vi "Update State Connections.vi"(8 "error in (no error)":errorcluster, 9 "connection list":T1[](array[typedef]), 10 "State":string, 11 "Channel Ref in":T2 format="%.0x") -> (0 "error out":errorcluster, 3 "Channel Ref out":T2=18446744073709551615 format="%.0x")   [LabVIEW 2017, in "Switch Scripting.lvlib"]
uses:
  Switch Scripting.lvlib
  <vilib>/NI Veristand/Custom Device API/Custom Device Item Ref.ctl
  Connection.ctl
  <vilib>/NI VeriStand/Custom Device API/Custom Device API.lvlib
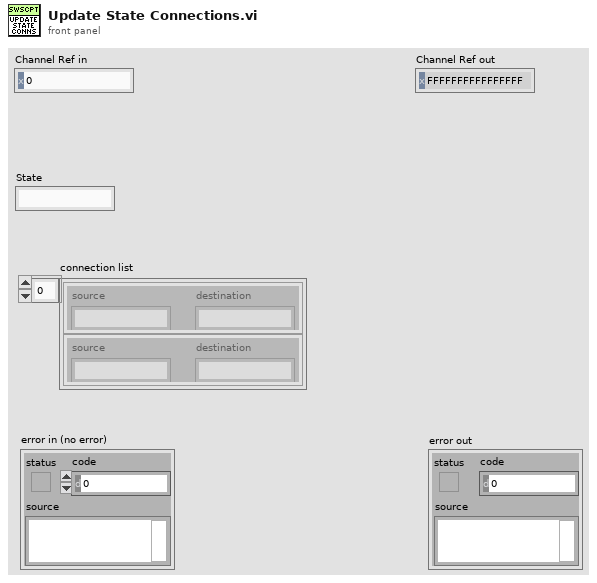
[diagram p1: front panel]
types:
  T1 = typedef "Switch Scripting.lvlib/Connection.ctl" = cluster{"source":string, "destination":string}
  T2 = typedef "Custom Device API.lvlib/Custom Device Item Ref.ctl" = u64
  T3 = typedef "Switch Scripting.lvlib/Routing State.ctl" = cluster{"name":string, "description":string, "value":i32, "connection list":T1[]}
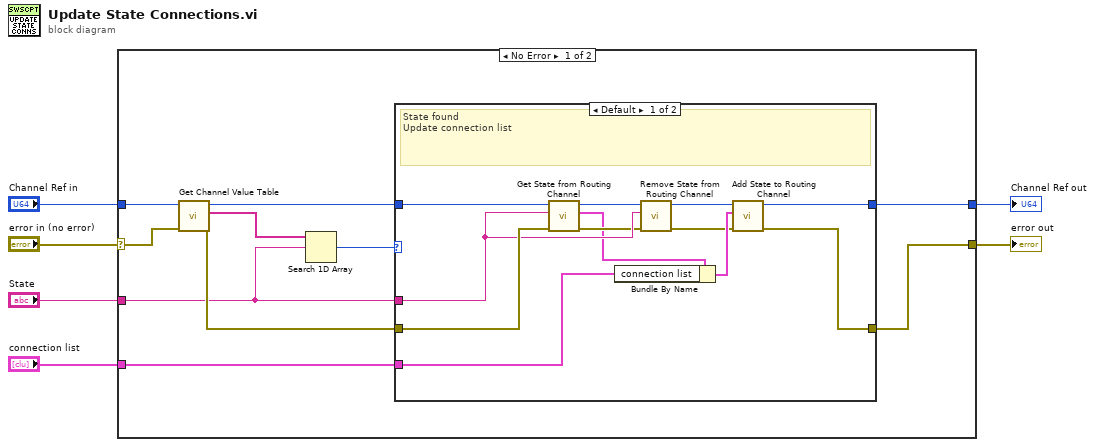
[diagram p0: block diagram]
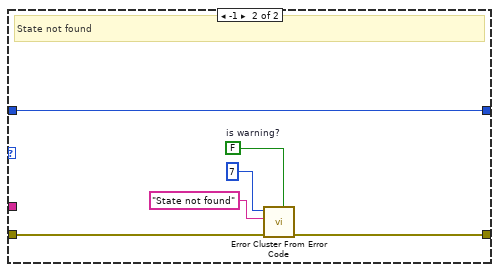
[diagram p2: hidden frame]
diagram:
  n1 = case shown="No Error" "error in (no error)" {
    selector: "error in (no error)" -> [w15 w36]
    tunnel: [w11 w36] -> w1
    tunnel: "Channel Ref in" -> [w16 w35]
    tunnel: [w12 w35] -> w2
    tunnel: "State" -> [w9 _]
    tunnel: "connection list" -> [w7 _]
    frame No Error {
      n2 = call "Get Channel Value Table.vi"("error in (no error)"=w15, "Channel Ref in"=w16) -> ("error out"=w13:errorcluster, "States"=w10:string[], "Channel Ref out"=w14:T2)  [unwired: 6 in, 1 out]
      n3 = Search 1D Array(1D array=w10, element=w9) -> (index of element=w8:i32)  [unwired: 1 in]
      n4 = case shown="Default" w8 {
        tunnel: w14 -> [w28 w29]
        tunnel: w13 -> [w27 w31]
        tunnel: [w24 w29] -> w12
        tunnel: [w25 w30] -> w11
        tunnel: w9 -> [w26 _]
        tunnel: w7 -> [w17 _]
        frame Default {
          # "State found\nUpdate connection list"
          n5 = call "Get State from Routing Channel.vi"("error in (no error)"=w27, "State"=w26, "Channel Ref in"=w28) -> ("error out"=w22:errorcluster, "Routing State"=w21:T3, "Channel Ref out"=w23:T2)  [unwired: 6 in]
          n6 = Bundle By Name(cluster=w21, "connection list"=w17) -> (w20:T3)
          n7 = call "Remove State from Routing Channel.vi"("error in (no error)"=w22, "State"=w26, "Channel Ref in"=w23) -> ("error out"=w18:errorcluster, "Channel Ref out"=w19:T2)  [unwired: 7 in]
          n8 = call "Add State to Routing Channel.vi"("error in (no error)"=w18, "Routing State"=w20, "Channel Ref in"=w19) -> ("error out"=w25:errorcluster, "Channel Ref out"=w24:T2)  [unwired: 7 in]
        }
        frame -1 {
          w33 = FALSE  # is warning?
          # "State not found"
          n9 = call <vilib>:"Error Cluster From Error Code.vi"("is warning? (False)"=w33, "error in (no error)"=w31, "error message (\"\")"="State not found" ("error message (\"\")"), "error code (0)"=7) -> ("error out"=w30:errorcluster)  [unwired: 5 in]
        }
      }
    }
    frame Error {
    }
  }
  "Channel Ref out" <- w2
  "error out" <- w1
